vi "Example of Arrays to JSON.vi"() -> ()   [LabVIEW 2017]
uses:
  2bd85c31-efc5-4a81-bc2d-e57801eae9cd.vi
  Variant to JSON Text.vi
panel:
  in  "Pretty Print?":bool
  out "Time per DBL":dbl[](array[numeric]) format="%#_3p"
  out "Time":dbl[](array[numeric]) format="%#_3p"
  out "<JSON>":string
  in  "Number in array":i32=10000
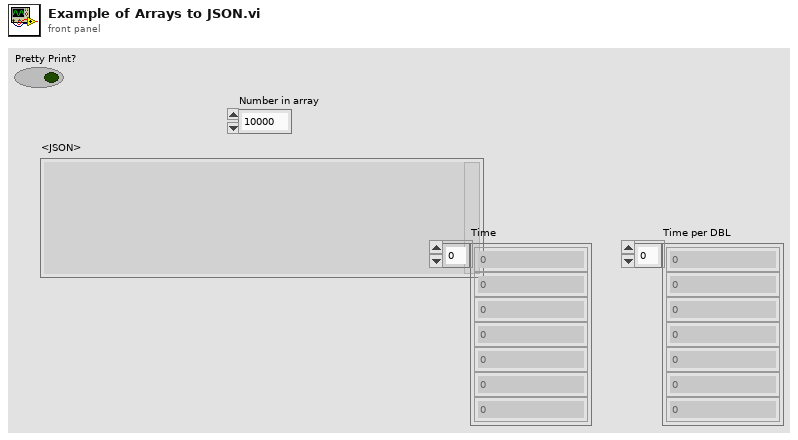
[diagram p1: front panel]
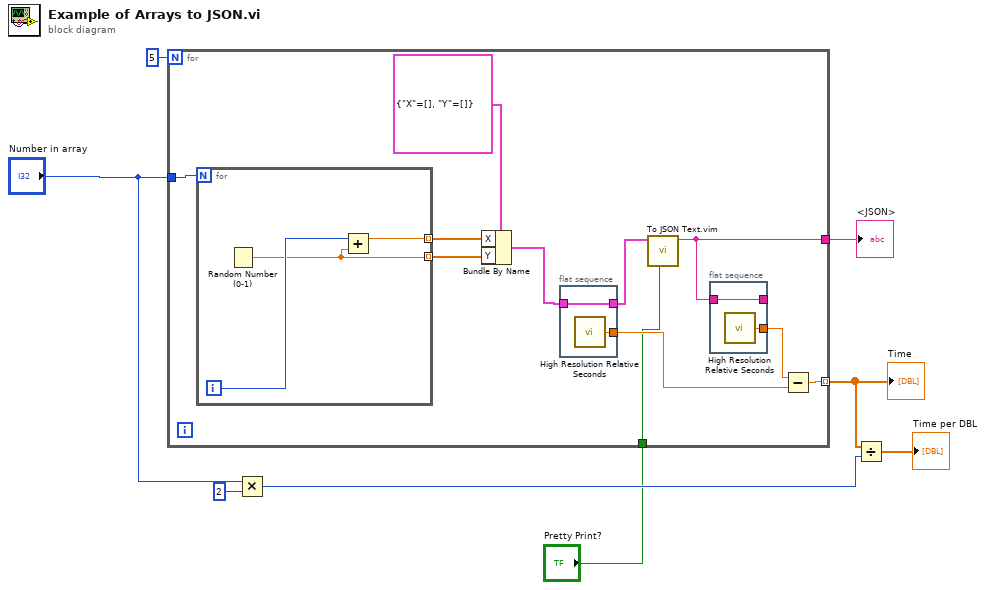
[diagram p0: block diagram]
diagram:
  n1 = for {
    N: 5 -> [_]
    tunnel: "Number in array" -> [w19]
    tunnel: [w13] -> w8
    tunnel: [w10] -> w6 mode=indexing
    tunnel: "Pretty Print?" -> [w9]
    n2 = for {
      N: w19 -> [_]
      tunnel: [w24] -> w17 mode=indexing
      tunnel: [w25] -> w18 mode=indexing
      i -> [w26]
      n3 = Random Number (0-1)() -> (number: 0 to 1=w24:dbl)
      n4 = Add(x=w26, y=w24) -> (x+y=w25:dbl)
    }
    n5 = Bundle By Name(cluster=cluster{"X":dbl[], "Y":dbl[]} {"X"=[], "Y"=[]}, "X"=w18, "Y"=w17) -> (w15:cluster{"X":dbl[], "Y":dbl[]})
    n6 = flat-sequence {
      tunnel: [w23] -> w14
      tunnel: w15 -> [w23]
      tunnel: [w22] -> w11
      frame #0 {
        n7 = call <vilib>:"High Resolution Relative Seconds.vi"() -> ("relative seconds"=w22:dbl)
      }
    }
    n8 = call "To JSON Text.vim"("Pretty Print?"=w9, "Anything"=w14) -> ("<JSON>"=w13:string)  [unwired: 8 in, 1 out]
    n9 = flat-sequence {
      tunnel: [w21] -> _
      tunnel: w13 -> [w21]
      tunnel: [w20] -> w12
      frame #0 {
        n10 = call <vilib>:"High Resolution Relative Seconds.vi"() -> ("relative seconds"=w20:dbl)
      }
    }
    n11 = Subtract(x=w12, y=w11) -> (x-y=w10:dbl)
  }
  "<JSON>" <- w8
  "Time" <- w6
  n12 = Multiply(x="Number in array", y=2) -> (x*y=w3:i32)
  n13 = Divide(x=w6, y=w3) -> (x/y=→"Time per DBL":dbl[])
